vi "Configure Trigger Event TSP Link.vi"(0 "VISA resource name":refnum<visa-resource-name>, 1 "Trigger Pulse Width (1E-6 S)":dbl=1e-06, 5 "Trigger Number (1)":i32=1, 7 "Trigger Mode (0: Bypass)":i32(ring) items=["Bypass", "Falling Edge", "Rising Edge", "Falling and Rising Edge", "Synchronous-A", "Synchronous", "Synchronous-M", "Rising-A", "Rising-M"], 9 "Event ID":string, 11 "error in (no error)":errorcluster) -> (4 "VISA resource name out":refnum<visa-resource-name>, 15 "error out":errorcluster)   [LabVIEW 2020, in "Keithley 2600 Series.lvlib"]
doc: "Configures the event that causes the synchronization line to assert a trigger.\n\n<b>Note:</b>\nThis VI is not available on the models 2604B, 2614B, and 2634B."
uses:
  <instrlib>/Keithley 2600 Series/Keithley 2600 Series.lvlib
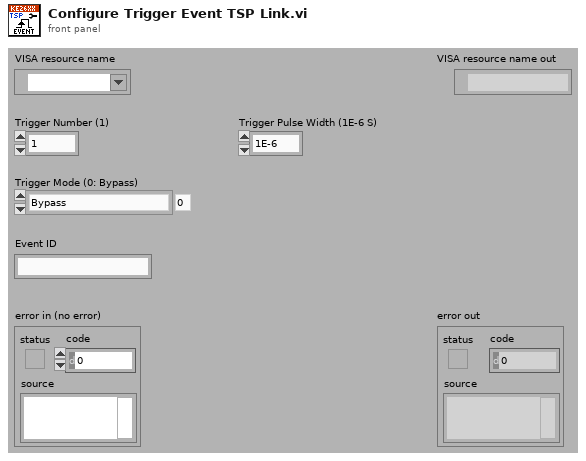
[diagram p1: front panel]
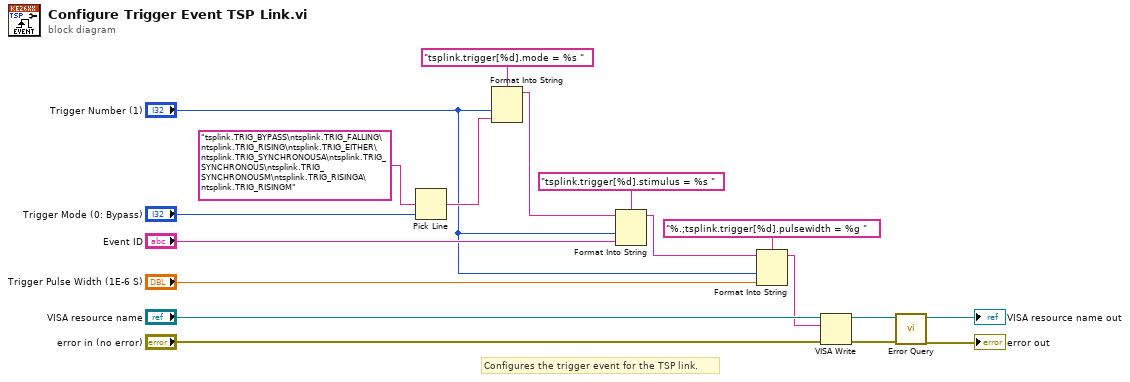
[diagram p0: block diagram]
diagram:
  # "Configures the trigger event for the TSP link."
  n1 = Pick Line(multi-line string="tsplink.TRIG_BYPASS\ntsplink.TRIG_FALLING\ntsplink.TRIG_RISING\ntsplink.TRIG_EITHER\ntsplink.TRIG_SYNCHRONOUSA\ntsplink.TRIG_SYNCHRONOUS\ntsplink.TRIG_SYNCHRONOUSM\ntsplink.TRIG_RISINGA\ntsplink.TRIG_RISINGM", line index="Trigger Mode (0: Bypass)") -> (output string=w14:string)  [unwired: 1 in]
  n2 = Format Into String(format string="tsplink.trigger[%d].mode = %s ", "Trigger Number (1)", w14) -> (resulting string=w7:string)  [unwired: 2 in, 1 out]
  n3 = Format Into String(format string="tsplink.trigger[%d].stimulus = %s ", initial string=w7, "Trigger Number (1)", "Event ID") -> (resulting string=w4:string)  [unwired: 1 in, 1 out]
  n4 = Format Into String(format string="%.;tsplink.trigger[%d].pulsewidth = %g ", initial string=w4, "Trigger Number (1)", "Trigger Pulse Width (1E-6 S)") -> (resulting string=w1:string)  [unwired: 1 in, 1 out]
  n5 = VISA Write(VISA resource name="VISA resource name", write buffer=w1, error in (no error)="error in (no error)") -> (VISA resource name out=w11:refnum<visa-resource-name>, error out=w10:errorcluster)  [unwired: 1 out]
  n6 = call <instrlib>:"Error Query.vi"("error in (no error)"=w10, "VISA resource name"=w11) -> ("error out"=→"error out":errorcluster, "VISA resource name out"=→"VISA resource name out":refnum<visa-resource-name>)  [unwired: 6 in, 2 out]
